vi "Init.vi"(8 "error in (no error)":errorcluster, 10 "Channel Index":i32, 11 "Group":refnum<class "Group DBL.lvclass">) -> (0 "error out":errorcluster, 3 "Channel out":refnum<class "Channel DBL.lvclass">)   [LabVIEW 2020, in "Vecto.lvlib" / "Channel DBL.lvclass"]
uses:
  Channel DBL.lvclass
  Group DBL/Group DBL.lvclass
  Channel DBL.lvclass/Channel DBL.ctl
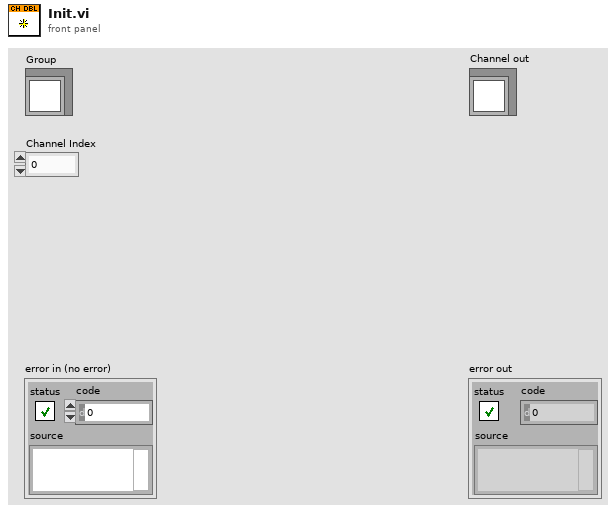
[diagram p1: front panel]
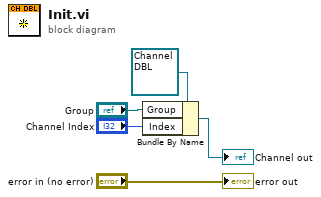
[diagram p0: block diagram]
diagram:
  n1 = Bundle By Name(cluster=refnum<class "Channel DBL.lvclass"> refnum ("Channel in"), "Group"="Group", "Index"="Channel Index") -> (→"Channel out":refnum<class "Channel DBL.lvclass">)
  "error out" <- "error in (no error)"
